vi "Demo Button and Alert server.vi"(8 "error in (no error)":errorcluster) -> (0 "error out":errorcluster)   [LabVIEW 2013]
doc: "reentrant"
uses:
  VIremote.llb/VIremoteEvent.ctl
  VIremote.llb/VIremoteFunction.ctl
panel:
  in  "next":bool
  in  "VIremoteEvent":T1
  in  "Slider iPad":i32(slide)=27 scale=0.0..100.0
  in  "A Slide can not be moved directly without emulation but you can change it via its popup.":i32(slide)=21 scale=0.0..50.0
  in  "Lights":bool
  in  "Test":bool
  in  "Message":string="My test message"
  out "Boolean":bool=TRUE
  # "Tap the button below to bring up an alert view with the above message. The \"Show Alert Message\" function return immediately (not waiting for the OK button)."
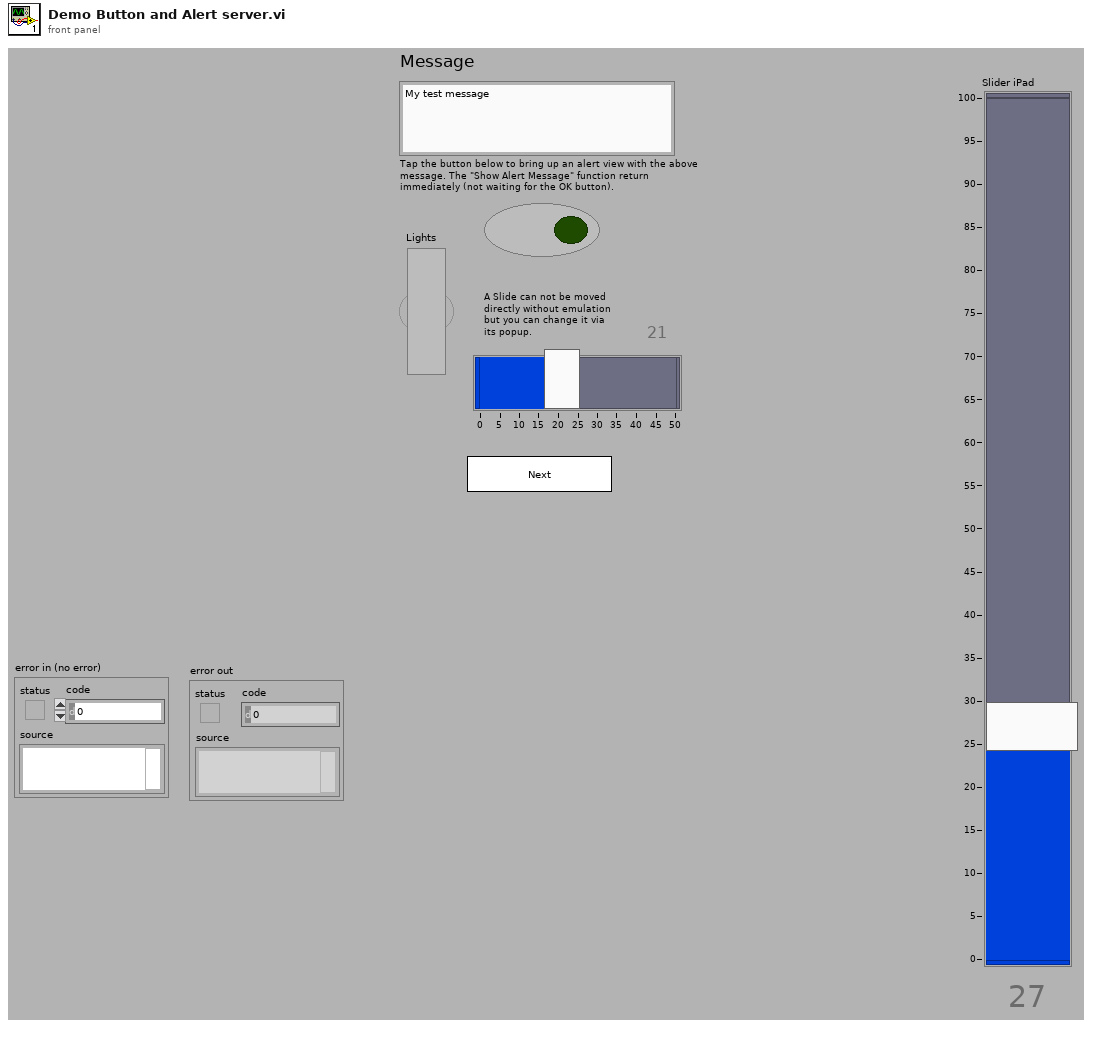
[diagram p1: front panel]
types:
  T1 = typedef "VIremoteEvent.ctl" = enum16{"No Event", "Connection Closed", "Navigate Back", "Enter Background", "Enter Foreground", "Portrait", "Portrait Upside Down", "Landscape Left", "Landscape Right"}
  T2 = typedef "VIremoteFunction.ctl" = enum16{"Do nothing", "Stop controller", "Close this connection", "Show info panel", "Set VI to control", "Set Accelerometer freq (Hz)", "Show Alert message", "Start Sound Input", "Stop Sound Input", "Set Volume (0-100)", "Set sound output Speaker", "Set sound output Receiver", "Play Sound", "Repeat Sound", "Stop Sound", "Pause Sound", "Resume Sound", "Set panel width of caller (320 or 480)", "Set Panel Size to Portrait", "Set Panel Size to Landscape", "Set Panel Size as Current Orientation", "Allow all UI Orientations", "Send user notification", "Disable Scrolling", "Normal Scrolling", "Page Scrolling", "Set Scroll Offset", "Page Indicator Position"}
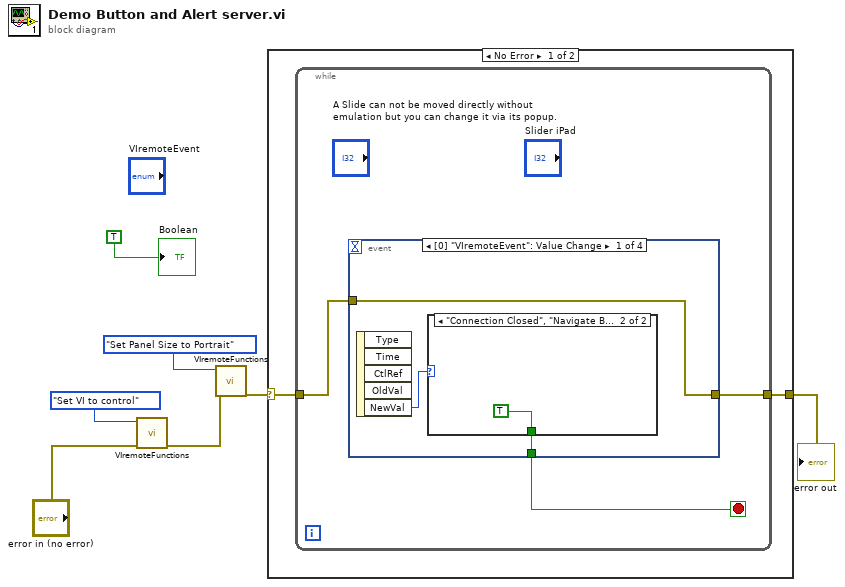
[diagram p0: block diagram]
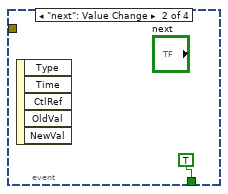
[diagram p3: hidden frame]
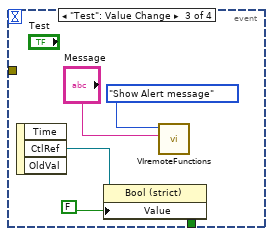
[diagram p4: hidden frame]
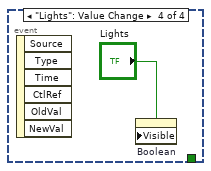
[diagram p5: hidden frame]
diagram:
  n1 = call "VIremoteFunctions.vi"("error in (no error)"="error in (no error)", "Function"=VIremoteFunction."Set VI to control") -> ("error out"=w4:errorcluster)  [unwired: 4 in, 5 out]
  n2 = call "VIremoteFunctions.vi"("error in (no error)"=w4, "Function"=VIremoteFunction."Set Panel Size to Portrait") -> ("error out"=w1:errorcluster)  [unwired: 4 in, 5 out]
  n3 = case shown="No Error" w1 {
    selector: w1 -> [w8 w23]
    tunnel: [w9 w23] -> w2
    frame No Error {
      n4 = while {
        tunnel: [w11] -> w9
        tunnel: w8 -> [w10]
        stop <- w12 stop-if-true
        n5 = event shown="[0] \"VIremoteEvent\": Value Change" {
          selector: _ -> [_ _ _ _]
          dyn-events: _ -> [_ _ _ _]
          timeout: _ -> [_ _ _ _]
          tunnel: [w15 TRUE ("status") _ _] -> w12
          tunnel: [w14 _ _ _] -> w11
          tunnel: w10 -> [w14 _ _ _]
          event Value Change {
            n6 = event-data() -> ("NewVal"=w13:T1)  [unwired: 5 out]
            n7 = case shown="\"Connection Closed\", \"Navigate Back\"" w13 {
              tunnel: [_ TRUE ("status")] -> w15
              frame "No Event", Default {
              }
              frame "Connection Closed", "Navigate Back" {
              }
            }
          }
          event "next": Value Change {
            n8 = event-data() -> ()  [unwired: 6 out]
          }
          event "Test": Value Change {
            n9 = event-data() -> ("CtlRef"=w18:refnum<vi>)  [unwired: 3 out]
            n10 = property class="Bool (strict)"(reference=w18, "Value"=FALSE ("+")) -> ()  [unwired: 1 in, 2 out]
            n11 = call "VIremoteFunctions.vi"("String in"="Message", "Function"=VIremoteFunction."Show Alert message") -> ()  [unwired: 4 in, 6 out]
          }
          event "Lights": Value Change {
            n12 = event-data() -> ()  [unwired: 7 out]
            n13 = property on="Boolean" class="Bool (strict)"("Visible"="Lights") -> ()  [unwired: 2 in, 2 out]
          }
        }
      }
    }
    frame Error {
    }
  }
  "error out" <- w2
  "Boolean" <- TRUE ("Boolean")
